vi "RT Engine.vi"(8 "Error In":errorcluster) -> ()   [LabVIEW 2019]
uses:
  <vilib>/NI/STM/TCP/TCP Connection Info.ctl
  <vilib>/NI/STM/SubVIs/MetaDataElement.ctl
  <vilib>/NI/STM/Connection Manager/TCP/TCP Connection Method.ctl
  PC/Event Mode.ctl
  <vilib>/NI/STM/Connection Manager/TCP/TCP Connection Properties.ctl
  <vilib>/NI/STM/TCP/TCP Read Options.ctl
  PC/PCsend RTrecv CMD.ctl
  TypeDef/TCP Cluster.ctl
  <vilib>/NI/STM/TCP/Write Meta Data (TCP Ref).vi
  <vilib>/NI/STM/TCP/Write Message (TCP).vi
  <vilib>/NI/STM/TCP/Write Meta Data (TCP Clst).vi
  <vilib>/NI/STM/TCP/Read Message (TCP).vi
  <vilib>/NI/STM/NI STM.lvlib
panel:
  out "conn?":bool
  out "SEND conn":T1
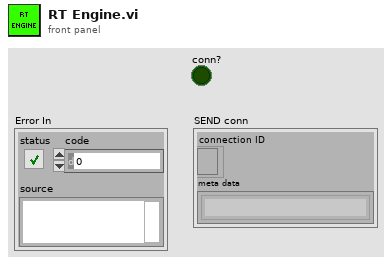
[diagram p1: front panel]
types:
  T1 = typedef "NI STM.lvlib/TCP Connection Info.ctl" = cluster{"connection ID":refnum<k5>, "meta data":T2[]}
  T2 = typedef "NI STM.lvlib/MetaDataElement.ctl" = string
  T3 = typedef "Event Mode.ctl" = enum16{"Init", "Get", "Set", "Destroy"}
  T4 = typedef "NI STM.lvlib/TCP Connection Method.ctl" = enum16{"Initialize", "Add Connection", "Set Properties", "Get Connection(s)", "Remove Connection", "Remove All Connections", "Get Connection Count"}
  T5 = typedef "NI STM.lvlib/TCP Connection Properties.ctl" = cluster{"Name":string, "Address":string, "Custom":string}
  T6 = typedef "NI STM.lvlib/TCP Read Options.ctl" = cluster{"ignore timeout error":bool, "timeout ms (1000)":i32}
  T7 = typedef "PCsend RTrecv CMD.ctl" = enum16{"ConnSettings", "Connect", "Stop", "Digital Outputs", "Analog Outputs", "Sweep Parameters", "Start Sweep", "Cal2RT", "Save Cal", "Load Cal"}
  T8 = typedef "TCP Cluster.ctl" = cluster{"Command":string, "FlattenedData":string}
  T9 = typedef "RTsend PCrecv CMD.ctl" = enum16{"Digital Inputs", "Connected?", "Data", "Data 2", "Cal2PC"}
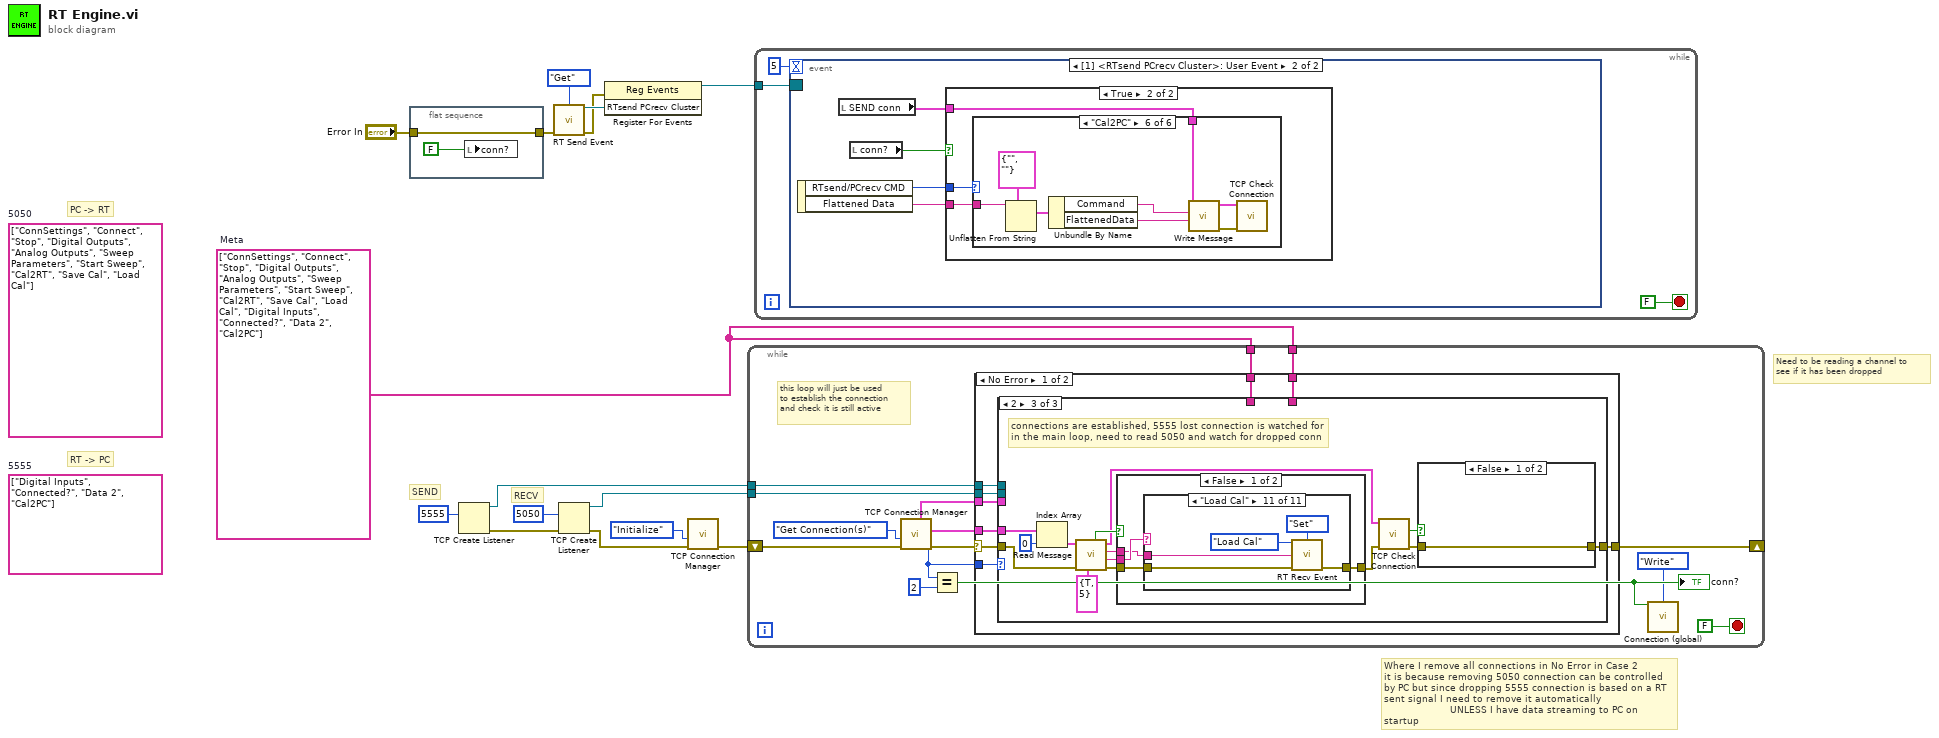
[diagram p0: block diagram]
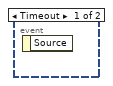
[diagram p2: hidden frame]
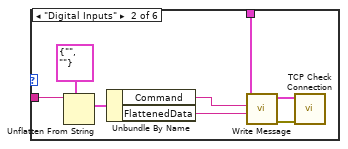
[diagram p5: hidden frame]
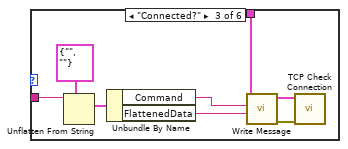
[diagram p6: hidden frame]
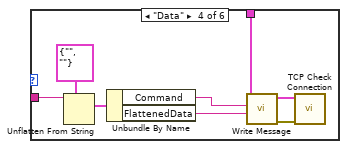
[diagram p7: hidden frame]
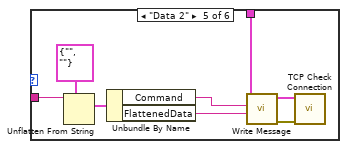
[diagram p8: hidden frame]
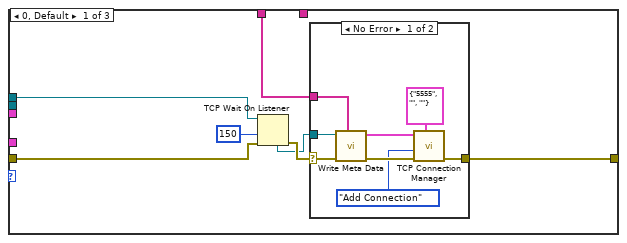
[diagram p9: hidden frame]
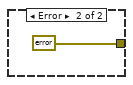
[diagram p10: hidden frame]
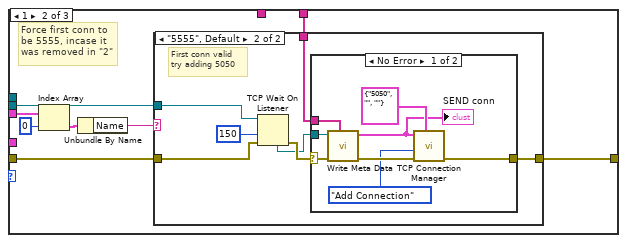
[diagram p11: hidden frame]
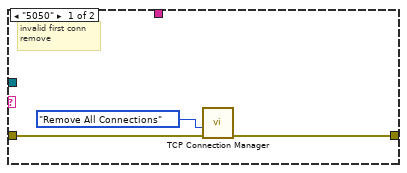
[diagram p12: hidden frame]
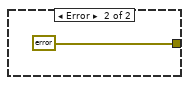
[diagram p13: hidden frame]
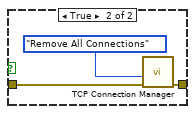
[diagram p14: hidden frame]
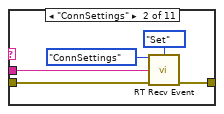
[diagram p17: hidden frame]
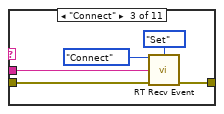
[diagram p18: hidden frame]
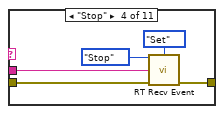
[diagram p19: hidden frame]
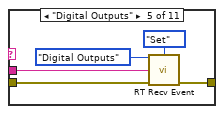
[diagram p20: hidden frame]
diagram:
  w1 = T2[] ["ConnSettings", "Connect", "Stop", "Digital Outputs", "Analog Outputs", "Sweep Parameters", "Start Sweep", "Cal2RT", "Save Cal", "Load Cal", "Digital Inputs", "Connected?", "Data 2", "Cal2PC"]  # Meta
  (unwired) T2[] ["Digital Inputs", "Connected?", "Data 2", "Cal2PC"]  # 5555
  (unwired) T2[] ["ConnSettings", "Connect", "Stop", "Digital Outputs", "Analog Outputs", "Sweep Parameters", "Start Sweep", "Cal2RT", "Save Cal", "Load Cal"]  # 5050
  # "PC -> RT"
  # "RT -> PC"
  # "Where I remove all connections in No Error in Case 2\nit is because removing 5050 connection can be controlled\nby PC but since dropping 5555 connection is based on a RT\nsent signal I need to remove it automatically\n                      UNLESS I have data streaming to PC on startup"
  # "Need to be reading a channel to\nsee if it has been dropped"
  # "SEND"
  # "RECV"
  n1 = flat-sequence {
    tunnel: "Error In" -> [w17]
    tunnel: [w17] -> w8
    frame #0 {
      n2 = local write "conn?"(FALSE ("stop")) -> ()
    }
  }
  n3 = TCP Create Listener(10:u16 5555 ("port")) -> (0:w6:errorcluster, 3:w5:refnum<k5>)  [unwired: 4 in, 1 out]
  n4 = call "RT Send Event.vi"("Mode"=Event_Mode."Get", "Error In"=w8) -> ("RTsend PCrecv Cluster"=w12:refnum<user-event>, "Error Out"=w11:errorcluster)  [unwired: 12 in]
  n5 = TCP Create Listener(8:w6, 10:u16 5050 ("port")) -> (0:w15:errorcluster, 3:w4:refnum<k5>)  [unwired: 3 in, 1 out]
  n6 = register-events(error in=w11, w12) -> (reference out=w10:refnum<event-registration>)  [unwired: 1 in, 1 out]
  n7 = call <vilib>:"TCP Connection Manager.vi"("error in"=w15, "method"=TCP_Connection_Method."Initialize") -> ("error out"=w13:errorcluster)  [unwired: 4 in, 5 out]
  n8 = while {
    shift-right: [w21] -> _
    shift-left: w13 -> [w32]
    tunnel: w1 -> [w29]
    tunnel: w5 -> [w26]
    tunnel: w4 -> [w25]
    tunnel: w1 -> [w20]
    stop <- FALSE stop-if-true
    # "this loop will just be used\nto establish the connection\nand check it is still active"
    n9 = call <vilib>:"TCP Connection Manager.vi"("error in"=w32, "method"=TCP_Connection_Method."Get Connection(s)") -> ("error out"=w30:errorcluster, "number of connections"=w22:i32, "all connections"=w24:T1[], "all properties"=w23:T5[])  [unwired: 4 in, 2 out]
    n10 = Equal?(x=w22, y=2) -> (x = y?=w19:bool)
    "conn?" <- w19
    n11 = case shown="No Error" w30 {
      selector: w30 -> [w41 _]
      tunnel: [w40 errorcluster {"status"=FALSE, "code"=0, "source"=""} ("t")] -> w21
      tunnel: w29 -> [w39 _]
      tunnel: w26 -> [w38 _]
      tunnel: w25 -> [w37 _]
      tunnel: w24 -> [w34 w162]
      tunnel: w23 -> [w35 _]
      tunnel: w22 -> [w36 _]
      tunnel: w20 -> [w33 _]
      frame No Error {
        n12 = case shown="2" w36 {
          tunnel: [w47 w65 w95] -> w40
          tunnel: w41 -> [w48 w58 w96]
          tunnel: w39 -> [_ w64 _]
          tunnel: w38 -> [w46 _ _]
          tunnel: w37 -> [_ w59 _]
          tunnel: w35 -> [_ w63 _]
          tunnel: w34 -> [_ _ w98]
          tunnel: w33 -> [w42 _ _]
          frame 0, Default {
            n13 = TCP Wait On Listener(8:w48, 9:150 ("timeout ms (wait forever: -1)"), 11:w46) -> (0:w44:errorcluster, 4:w43:refnum<k5>)  [unwired: 1 in, 3 out]
            n14 = case shown="No Error" w44 {
              selector: w44 -> [w56 _]
              tunnel: [w54 errorcluster {"status"=FALSE, "code"=0, "source"=""} ("error constant")] -> w47
              tunnel: w43 -> [w53 _]
              tunnel: w42 -> [w51 _]
              frame No Error {
                n15 = call-poly <vilib>:"Write Meta Data.vi"("meta data"=w51, "error in"=w56, "connection ID"=w53) -> ("error out"=w55:errorcluster, "connection info out"=w49:T1)  [unwired: 7 in]
                n16 = call <vilib>:"TCP Connection Manager.vi"("properties in"=T5 {"Name"="5555", "Address"="", "Custom"=""}, "error in"=w55, "method"=TCP_Connection_Method."Add Connection", "connection in"=w49) -> ("error out"=w54:errorcluster)  [unwired: 2 in, 5 out]
              }
              frame Error {
              }
            }
          }
          frame 1 {
            # "Force first conn to\nbe 5555, incase it\nwas removed in \"2\""
            n17 = Index Array(array=w63, index=0) -> (element=w62:T5)
            n18 = Unbundle By Name(w62) -> ("Name"=w60:string)
            n19 = case shown="\"5555\", Default" w60 {
              tunnel: [w66 w75] -> w65
              tunnel: w64 -> [_ w74]
              tunnel: w58 -> [w67 w70]
              tunnel: w59 -> [_ w69]
              frame "5050" {
                # "invalid first conn\nremove"
                n20 = call <vilib>:"TCP Connection Manager.vi"("error in"=w67, "method"=TCP_Connection_Method."Remove All Connections") -> ("error out"=w66:errorcluster)  [unwired: 4 in, 5 out]
              }
              frame "5555", Default {
                # "First conn valid\ntry adding 5050"
                n21 = TCP Wait On Listener(8:w70, 9:150 ("timeout ms (wait forever: -1)"), 11:w69) -> (0:w72:errorcluster, 4:w71:refnum<k5>)  [unwired: 1 in, 3 out]
                n22 = case shown="No Error" w72 {
                  selector: w72 -> [w83 _]
                  tunnel: [w81 errorcluster {"status"=FALSE, "code"=0, "source"=""} ("error constant")] -> w75
                  tunnel: w71 -> [w80 _]
                  tunnel: w74 -> [w78 _]
                  frame No Error {
                    n23 = call-poly <vilib>:"Write Meta Data.vi"("meta data"=w78, "error in"=w83, "connection ID"=w80) -> ("error out"=w82:errorcluster, "connection info out"=w76:T1)  [unwired: 7 in]
                    "SEND conn" <- w76
                    n24 = call <vilib>:"TCP Connection Manager.vi"("properties in"=T5 {"Name"="5050", "Address"="", "Custom"=""}, "error in"=w82, "method"=TCP_Connection_Method."Add Connection", "connection in"=w76) -> ("error out"=w81:errorcluster)  [unwired: 2 in, 5 out]
                  }
                  frame Error {
                  }
                }
              }
            }
          }
          frame 2 {
            # "connections are established, 5555 lost connection is watched for\nin the main loop, need to read 5050 and watch for dropped conn"
            n25 = Index Array(array=w98, index=0) -> (element=w94:T1)
            n26 = call-poly <vilib>:"Read Message.vi"("options"=T6 {"ignore timeout error"=TRUE, "timeout ms (1000)"=5}, "error in"=w96, "connection info in"=w94) -> ("error out"=w92:errorcluster, "name"=w91:T2, "data string"=w90:string, "connection info out"=w89:T1, "timed out?"=w93:bool)  [unwired: 3 in, 1 out]
            n27 = case shown="False" w93 {
              tunnel: w92 -> [w105 w159]
              tunnel: [w104 w159] -> w88
              tunnel: w91 -> [w106 _]
              tunnel: w90 -> [w103 _]
              frame False {
                n28 = case shown="\"Load Cal\"" w106 {
                  selector: w106 -> [w107 _ _ _ _ _ _ _ _ _ _]
                  tunnel: w105 -> [w108 w112 w117 w122 w127 w132 w137 w142 w147 w152 w157]
                  tunnel: [w108 w111 w115 w121 w126 w130 w135 w140 w145 w150 w155] -> w104
                  tunnel: w103 -> [_ w110 w116 w120 w125 w131 w136 w141 w146 w151 w156]
                  frame Default {
                    n29 = disable-structure shown="Disabled" {
                      disable-tunnel: w107 -> [_ _]
                      frame Disabled {
                      }
                      frame Enabled {
                      }
                    }
                  }
                  frame "ConnSettings" {
                    n30 = call "RT Recv Event.vi"("PCsend/RTrecv CMD"=PCsend_RTrecv_CMD."ConnSettings", "Mode"=Event_Mode."Set", "Flattened Data"=w110, "Error In"=w112) -> ("Error Out"=w111:errorcluster)  [unwired: 10 in, 1 out]
                  }
                  frame "Connect" {
                    n31 = call "RT Recv Event.vi"("PCsend/RTrecv CMD"=PCsend_RTrecv_CMD."Connect", "Mode"=Event_Mode."Set", "Flattened Data"=w116, "Error In"=w117) -> ("Error Out"=w115:errorcluster)  [unwired: 10 in, 1 out]
                  }
                  frame "Stop" {
                    n32 = call "RT Recv Event.vi"("PCsend/RTrecv CMD"=PCsend_RTrecv_CMD."Stop", "Mode"=Event_Mode."Set", "Flattened Data"=w120, "Error In"=w122) -> ("Error Out"=w121:errorcluster)  [unwired: 10 in, 1 out]
                  }
                  frame "Digital Outputs" {
                    n33 = call "RT Recv Event.vi"("PCsend/RTrecv CMD"=PCsend_RTrecv_CMD."Digital Outputs", "Mode"=Event_Mode."Set", "Flattened Data"=w125, "Error In"=w127) -> ("Error Out"=w126:errorcluster)  [unwired: 10 in, 1 out]
                  }
                  frame "Analog Outputs" {
                    n34 = call "RT Recv Event.vi"("PCsend/RTrecv CMD"=PCsend_RTrecv_CMD."Analog Outputs", "Mode"=Event_Mode."Set", "Flattened Data"=w131, "Error In"=w132) -> ("Error Out"=w130:errorcluster)  [unwired: 10 in, 1 out]
                  }
                  frame "Sweep Parameters" {
                    n35 = call "RT Recv Event.vi"("PCsend/RTrecv CMD"=PCsend_RTrecv_CMD."Sweep Parameters", "Mode"=Event_Mode."Set", "Flattened Data"=w136, "Error In"=w137) -> ("Error Out"=w135:errorcluster)  [unwired: 10 in, 1 out]
                  }
                  frame "Start Sweep" {
                    n36 = call "RT Recv Event.vi"("PCsend/RTrecv CMD"=PCsend_RTrecv_CMD."Start Sweep", "Mode"=Event_Mode."Set", "Flattened Data"=w141, "Error In"=w142) -> ("Error Out"=w140:errorcluster)  [unwired: 10 in, 1 out]
                  }
                  frame "Cal2RT" {
                    n37 = call "RT Recv Event.vi"("PCsend/RTrecv CMD"=PCsend_RTrecv_CMD."Cal2RT", "Mode"=Event_Mode."Set", "Flattened Data"=w146, "Error In"=w147) -> ("Error Out"=w145:errorcluster)  [unwired: 10 in, 1 out]
                  }
                  frame "Save Cal" {
                    n38 = call "RT Recv Event.vi"("PCsend/RTrecv CMD"=PCsend_RTrecv_CMD."Save Cal", "Mode"=Event_Mode."Set", "Flattened Data"=w151, "Error In"=w152) -> ("Error Out"=w150:errorcluster)  [unwired: 10 in, 1 out]
                  }
                  frame "Load Cal" {
                    n39 = call "RT Recv Event.vi"("PCsend/RTrecv CMD"=PCsend_RTrecv_CMD."Load Cal", "Mode"=Event_Mode."Set", "Flattened Data"=w156, "Error In"=w157) -> ("Error Out"=w155:errorcluster)  [unwired: 10 in, 1 out]
                  }
                }
              }
              frame True {
              }
            }
            n40 = call <vilib>:"TCP Check Connection.vi"("error in"=w88, "connection in"=w89) -> ("error out"=w87:errorcluster, "disconnected?"=w86:bool)  [unwired: 7 in, 1 out]
            n41 = case shown="False" w86 {
              tunnel: w87 -> [w99 w101]
              tunnel: [w99 w100] -> w95
              frame False {
              }
              frame True {
                n42 = call <vilib>:"TCP Connection Manager.vi"("error in"=w101, "method"=TCP_Connection_Method."Remove All Connections") -> ("error out"=w100:errorcluster)  [unwired: 4 in, 5 out]
              }
            }
          }
        }
      }
      frame Error {
        n43 = for {
          tunnel: w162 -> [w166] mode=indexing
          tunnel: errorcluster {"status"=FALSE, "code"=0, "source"=""} ("t") -> [w165]
          tunnel: [w164] -> w160
          n44 = call <vilib>:"TCP Check Connection.vi"("error in"=w165, "connection in"=w166) -> ("error out"=w164:errorcluster)  [unwired: 7 in, 2 out]
        }
        n45 = call <vilib>:"Clear Errors.vi"("error in (no error)"=w160) -> ()  [unwired: 5 in, 2 out]
      }
    }
    n46 = call "Connection (global).vi"("PC Connected In"=w19, "Mode"=enum16{"Read", "Write"}."Write") -> ()  [unwired: 13 in, 1 out]
  }
  n47 = while {
    tunnel: w10 -> [w168]
    stop <- FALSE stop-if-true
    n48 = event shown="[1] <RTsend PCrecv Cluster>: User Event" {
      selector: w168 -> [_ _]
      dyn-events: _ -> [_ _]
      timeout: 5 -> [_ _]
      event Timeout {
        n49 = event-data() -> ()  [unwired: 1 in, 1 out]
      }
      event User Event {
        n50 = event-data() -> ("RTsend/PCrecv CMD"=w171:T9, "Flattened Data"=w173:string)  [unwired: 1 in]
        n51 = local read "SEND conn"() -> (w170:T1)
        n52 = local read "conn?"() -> (w172:bool)
        n53 = case shown="True" w172 {
          tunnel: w173 -> [_ w175]
          tunnel: w171 -> [_ w176]
          tunnel: w170 -> [_ w174]
          frame False {
          }
          frame True {
            n54 = case shown="\"Cal2PC\"" w176 {
              tunnel: w174 -> [_ w180 w188 w196 w204 w212]
              tunnel: w175 -> [_ w179 w187 w195 w203 w211]
              frame Default {
              }
              frame "Digital Inputs" {
                n55 = Unflatten From String(type=T8 {"Command"="", "FlattenedData"=""}, binary string=w179) -> (value=w182:T8)  [unwired: 3 in, 2 out]
                n56 = Unbundle By Name(w182) -> ("Command"=w184:string, "FlattenedData"=w183:string)
                n57 = call-poly <vilib>:"Write Message.vi"("data"=w183, "name"=w184, "connection info in"=w180) -> ("error out"=w178:errorcluster, "connection info out"=w177:T1)  [unwired: 7 in]
                n58 = call <vilib>:"TCP Check Connection.vi"("error in"=w178, "connection in"=w177) -> ()  [unwired: 7 in, 3 out]
              }
              frame "Connected?" {
                n59 = Unflatten From String(type=T8 {"Command"="", "FlattenedData"=""}, binary string=w187) -> (value=w190:T8)  [unwired: 3 in, 2 out]
                n60 = Unbundle By Name(w190) -> ("Command"=w192:string, "FlattenedData"=w191:string)
                n61 = call-poly <vilib>:"Write Message.vi"("data"=w191, "name"=w192, "connection info in"=w188) -> ("error out"=w185:errorcluster, "connection info out"=w186:T1)  [unwired: 7 in]
                n62 = call <vilib>:"TCP Check Connection.vi"("error in"=w185, "connection in"=w186) -> ()  [unwired: 7 in, 3 out]
              }
              frame "Data" {
                n63 = Unflatten From String(type=T8 {"Command"="", "FlattenedData"=""}, binary string=w195) -> (value=w198:T8)  [unwired: 3 in, 2 out]
                n64 = Unbundle By Name(w198) -> ("Command"=w200:string, "FlattenedData"=w199:string)
                n65 = call-poly <vilib>:"Write Message.vi"("data"=w199, "name"=w200, "connection info in"=w196) -> ("error out"=w193:errorcluster, "connection info out"=w194:T1)  [unwired: 7 in]
                n66 = call <vilib>:"TCP Check Connection.vi"("error in"=w193, "connection in"=w194) -> ()  [unwired: 7 in, 3 out]
              }
              frame "Data 2" {
                n67 = Unflatten From String(type=T8 {"Command"="", "FlattenedData"=""}, binary string=w203) -> (value=w206:T8)  [unwired: 3 in, 2 out]
                n68 = Unbundle By Name(w206) -> ("Command"=w208:string, "FlattenedData"=w207:string)
                n69 = call-poly <vilib>:"Write Message.vi"("data"=w207, "name"=w208, "connection info in"=w204) -> ("error out"=w201:errorcluster, "connection info out"=w202:T1)  [unwired: 7 in]
                n70 = call <vilib>:"TCP Check Connection.vi"("error in"=w201, "connection in"=w202) -> ()  [unwired: 7 in, 3 out]
              }
              frame "Cal2PC" {
                n71 = Unflatten From String(type=T8 {"Command"="", "FlattenedData"=""}, binary string=w211) -> (value=w214:T8)  [unwired: 3 in, 2 out]
                n72 = Unbundle By Name(w214) -> ("Command"=w216:string, "FlattenedData"=w215:string)
                n73 = call-poly <vilib>:"Write Message.vi"("data"=w215, "name"=w216, "connection info in"=w212) -> ("error out"=w209:errorcluster, "connection info out"=w210:T1)  [unwired: 7 in]
                n74 = call <vilib>:"TCP Check Connection.vi"("error in"=w209, "connection in"=w210) -> ()  [unwired: 7 in, 3 out]
              }
            }
          }
        }
      }
    }
  }
